vi "Match.vi"(8 "error in (no error)":errorcluster, 10 "Match String":string, 11 "JSON Lexer in":refnum<class "JSON Lexer.lvclass">) -> (0 "error out":errorcluster, 1 "EOF":bool, 2 "Matched?":bool, 3 "JSON Lexer out":refnum<class "JSON Lexer.lvclass">)   [LabVIEW 2013, in "JKI JSON Serialization.lvlib" / "JSON Lexer.lvclass"]
uses:
  JSON Lexer.lvclass
  JSON Lexer.lvclass/JSON Lexer.ctl
  <vilib>/addons/_JKI.lib/Unicode/UTF-8 String/UTF-8 String.lvclass/UTF-8 String.ctl
  <vilib>/addons/_JKI.lib/Unicode/UTF-8 String/UTF-8 String.lvclass
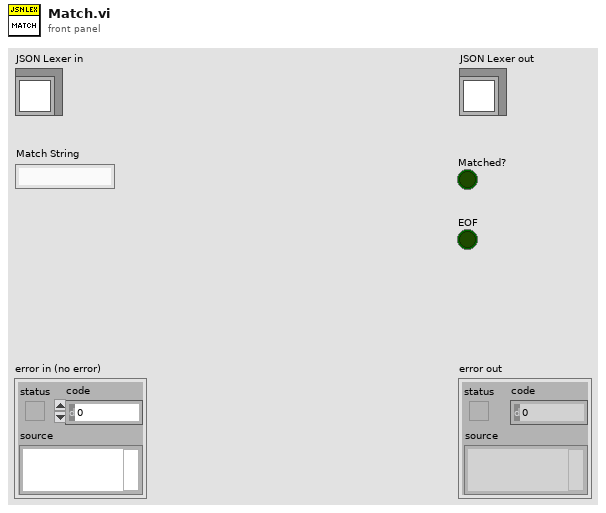
[diagram p1: front panel]
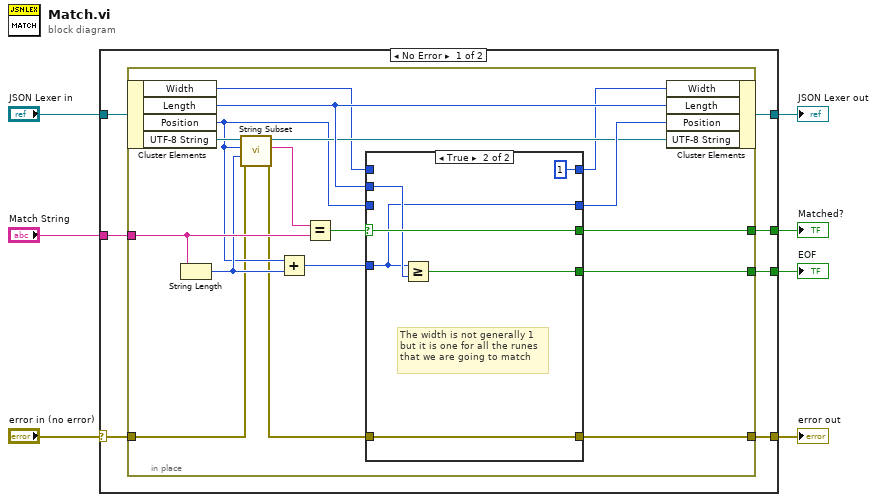
[diagram p0: block diagram]
diagram:
  n1 = case shown="No Error" "error in (no error)" {
    selector: "error in (no error)" -> [w11 w43]
    tunnel: [w14 w43] -> w6
    tunnel: [w8 w42] -> w4
    tunnel: "JSON Lexer in" -> [w9 w42]
    tunnel: "Match String" -> [w10 _]
    tunnel: [w13 _] -> w2
    tunnel: [w12 _] -> w1
    frame No Error {
      n2 = in-place {
        in-place-border: [w31] -> w14
        in-place-border: [w30] -> w13
        in-place-border: [w27] -> w12
        in-place-border: w11 -> [w16]
        in-place-border: w10 -> [w26]
        n3 = in-place-cluster #1(w9) -> ("Width"=w19:i32, "Length"=w24:i32, "Position"=w17:i32, "UTF-8 String"=w23:refnum<class "UTF-8 String.lvclass">)
        n4 = String Length(string=w26) -> (length=w22:i32)
        n5 = call <vilib>:"String Subset.vi"("error in (no error)"=w16, "Length in Bytes (0)"=w22, "Byte Offset (0)"=w17, "UTF8 in"=w23) -> ("error out"=w15:errorcluster, "String Subset"=w21:string, "UTF8 out"=w20:refnum<class "UTF-8 String.lvclass">)  [unwired: 5 in]
        n6 = Add(x=w17, y=w22) -> (x+y=w28:i32)
        n7 = Equal?(x=w21, y=w26) -> (x = y?=w29:bool)
        n8 = case shown="True" w29 {
          selector: w29 -> [w35 w41]
          tunnel: [w34 w38] -> w31
          tunnel: [w35 w41] -> w30
          tunnel: w28 -> [_ w37]
          tunnel: w24 -> [_ w40]
          tunnel: [_ w39] -> w27
          tunnel: w15 -> [w34 w38]
          tunnel: [w33 w37] -> w25
          tunnel: w17 -> [w33 _]
          tunnel: w19 -> [w32 _]
          tunnel: [w32 1 ("Width")] -> w18
          frame False {
          }
          frame True {
            # "The width is not generally 1\nbut it is one for all the runes\nthat we are going to match"
            n9 = Greater Or Equal?(x=w37, y=w40) -> (x >= y?=w39:bool)
          }
        }
        n10 = in-place-cluster #1("Width"=w18, "Length"=w24, "Position"=w25, "UTF-8 String"=w20) -> (w8:refnum<class "JSON Lexer.lvclass">)
      }
    }
    frame Error {
    }
  }
  "error out" <- w6
  "JSON Lexer out" <- w4
  "Matched?" <- w2
  "EOF" <- w1
